vi "SUB-BLE SCAN.vi"(5 "Port-set 1":refnum<visa-resource-name>="COM8" caption="COM port") -> (0 "Device Name":string, 1 "Connection Status":T1={"MAC Address"="D9:2F:10:92:34:F2", "cnx handle"=0, "cnx flags"=5, "Address Type"=1, "Connection Interval (ms)"=15, "Timeout(ms)"=1000, "Latency"=0, "bonding handle"=255} {"Address Type" items=["Public", "Random"]}, 2 "Connected":bool)   [LabVIEW 2015]
doc: "Use this template to create an application that executes repeatedly until you click the Stop button. This template polls the state of the Stop button and does not use events. Use the Top-Level Application template (not available in the Base package) to create a single-loop application with event handling."
uses:
  Lib_Bled112 toolkit/type_def/connection_status_bundle.ctl
  Lib_Bled112 toolkit/type_def/address_type.ctl
panel:
  out "Discovery":bool
  out "conn flag":bool
  out "Handle table":string[][](array[string])
  out "Address Type":enum16{"Public", "Random"}(ring)=enum."Random"
  out "MAC Address":string="D9:2F:10:92:34:F2"
  in  "Cancel":bool
  in  "Connection":bool
  in  "새로 검색":bool
  out "Start Search":bool caption="검색 시작"
  out "Complete":bool
  in  "Device List":i32(listbox)=2
  out "Scanning":bool
  # "Device Select"
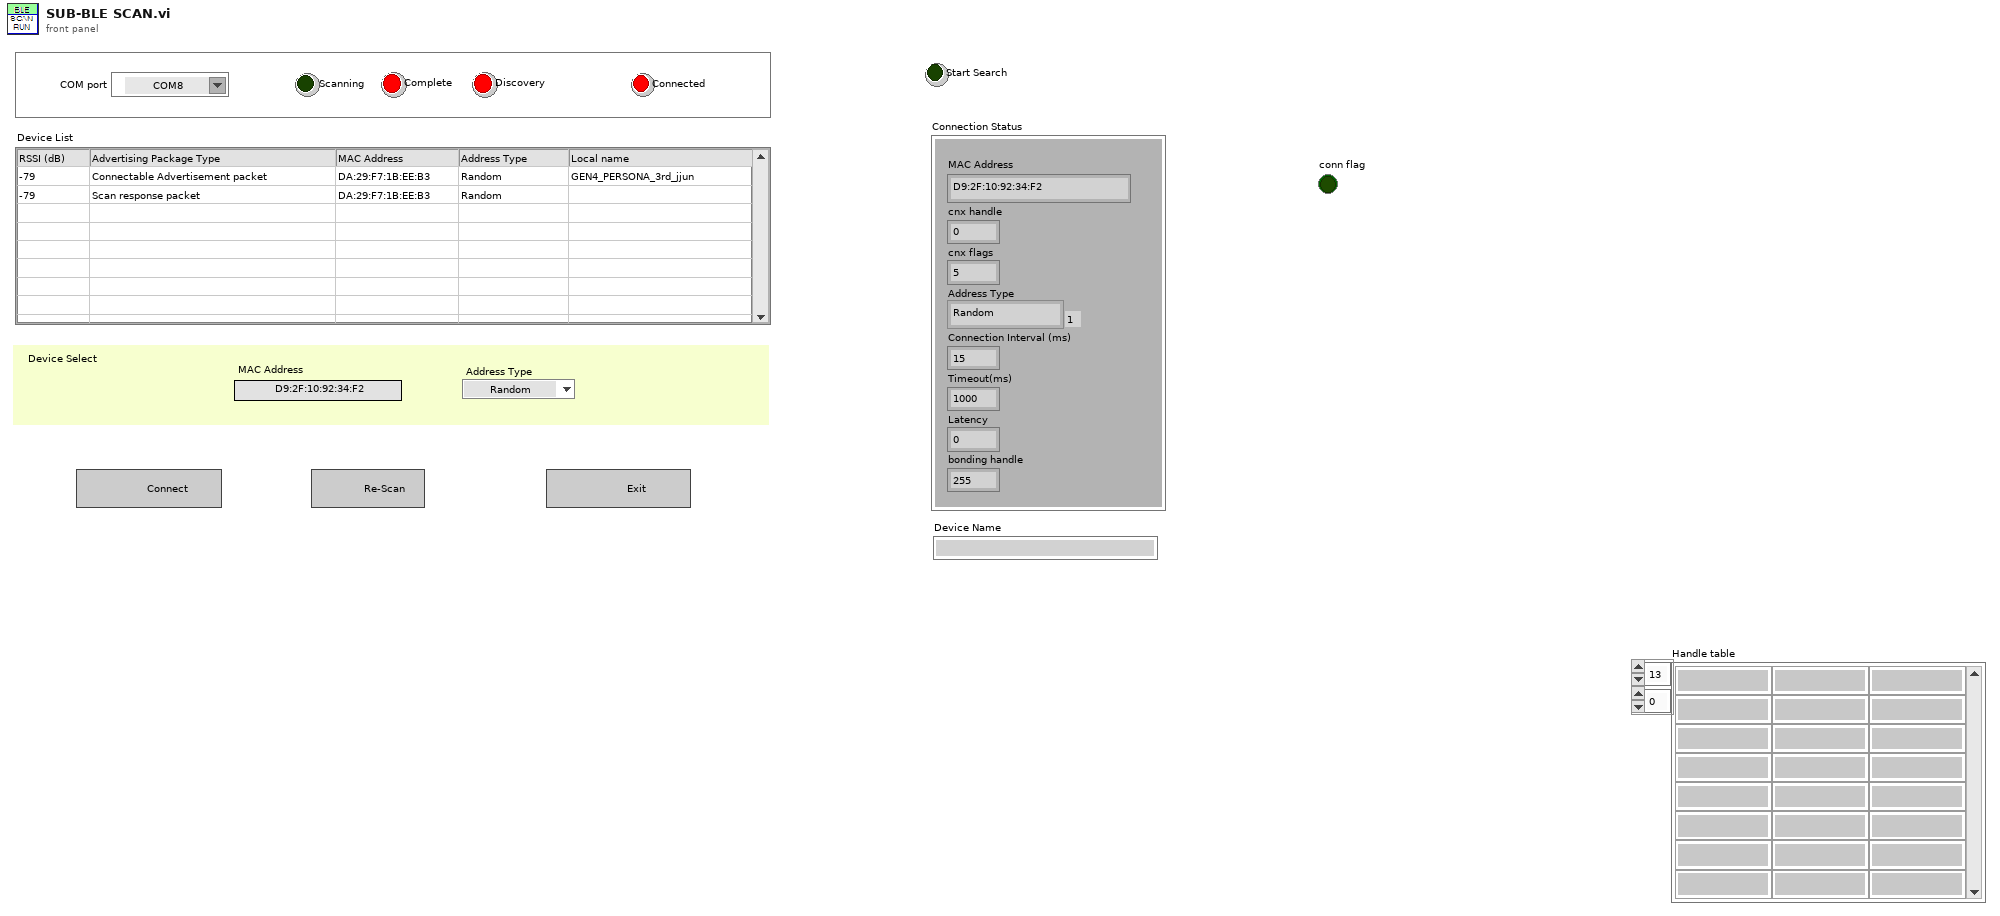
[diagram p1: front panel]
types:
  T1 = typedef "connection_status_bundle.ctl" = cluster{"MAC Address":string, "cnx handle":u8, "cnx flags":u8, "Address Type":T2, "Connection Interval (ms)":u16, "Timeout(ms)":u16, "Latency":u16, "bonding handle":u8}
  T2 = typedef "address_type.ctl" = u8
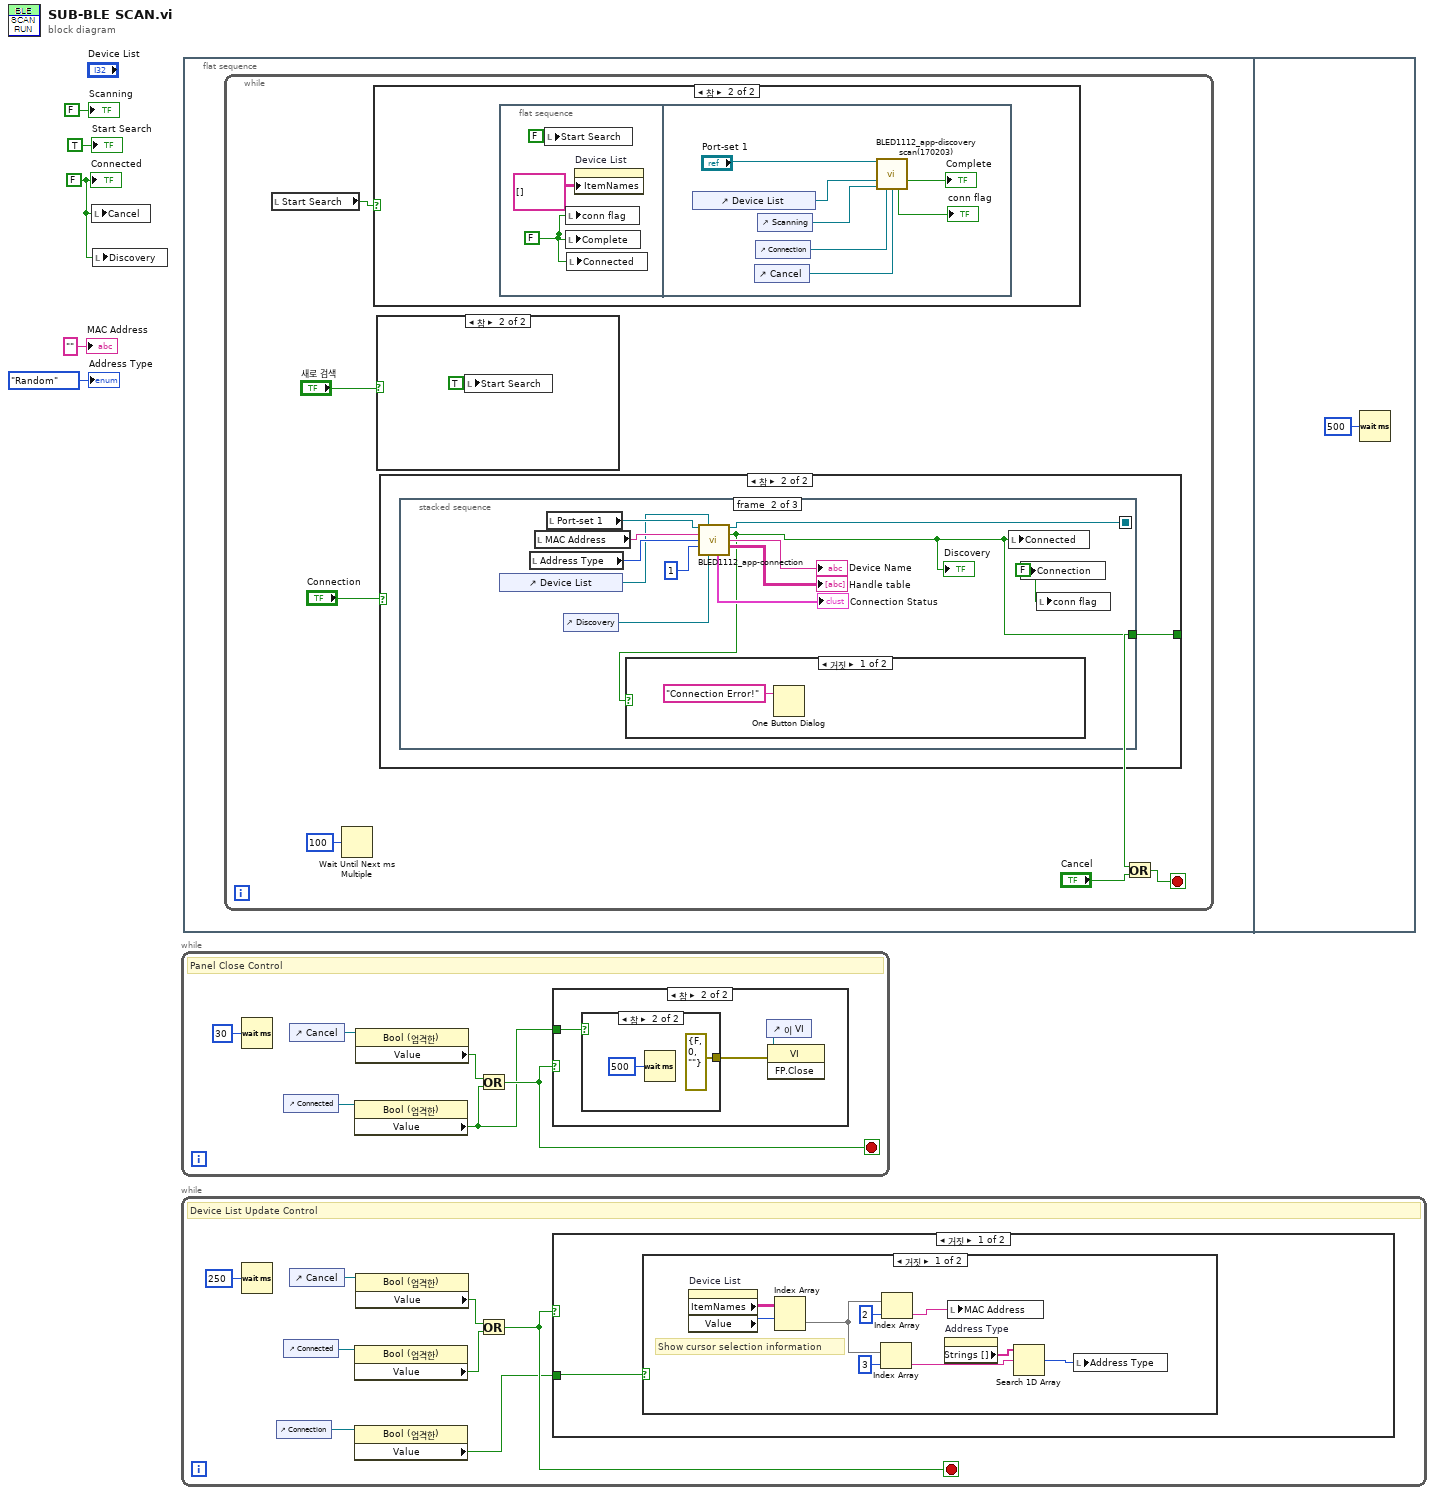
[diagram p0: block diagram]
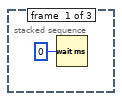
[diagram p7: hidden frame]
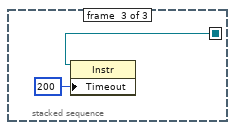
[diagram p9: hidden frame]
diagram:
  w1 = FALSE ("Connected")
  n1 = local write "Cancel"(w1) -> ()
  n2 = local write "Discovery"(w1) -> ()
  n3 = while {
    stop <- w7 stop-if-true
    # "Panel Close Control"
    n4 = Wait (ms)(milliseconds to wait=u32 30 ("대기 시간(ms)")) -> ()  [unwired: 1 out]
    n5 = control-ref of="Connected"() -> (w9:refnum<vi>)
    n6 = control-ref of="Cancel"() -> (w10:refnum<vi>)
    n7 = property class="Bool (엄격한)"(reference=w9) -> ("Value"=w6:bool)  [unwired: 1 in, 2 out]
    n8 = property class="Bool (엄격한)"(reference=w10) -> ("Value"=w8:bool)  [unwired: 1 in, 2 out]
    n9 = Or(x=w8, y=w6) -> (x .or. y?=w7:bool)
    n10 = case shown="참" w7 {
      tunnel: w6 -> [_ w13]
      frame False {
      }
      frame True {
        n11 = case shown="참" w13 {
          tunnel: [_ errorcluster {"status"=FALSE, "code"=0, "source"=""} ("에러 상수")] -> w12
          frame False {
          }
          frame True {
            n12 = Wait (ms)(milliseconds to wait=u32 500 ("대기 시간(ms)")) -> ()  [unwired: 1 out]
          }
        }
        n13 = control-ref of="이 VI"() -> (w14:refnum<vi>)
        n14 = invoke class="VI" method="FP.Close"(reference=w14, error in=w12) -> ()  [unwired: 1 in, 3 out]
      }
    }
  }
  n15 = while {
    stop <- w20 stop-if-true
    # "Device List Update Control"
    n16 = Wait (ms)(milliseconds to wait=u32 250 ("대기 시간(ms)")) -> ()  [unwired: 1 out]
    n17 = control-ref of="Connection"() -> (w18:refnum<vi>)
    n18 = control-ref of="Connected"() -> (w22:refnum<vi>)
    n19 = control-ref of="Cancel"() -> (w23:refnum<vi>)
    n20 = property class="Bool (엄격한)"(reference=w22) -> ("Value"=w19:bool)  [unwired: 1 in, 2 out]
    n21 = property class="Bool (엄격한)"(reference=w18) -> ("Value"=w17:bool)  [unwired: 1 in, 2 out]
    n22 = property class="Bool (엄격한)"(reference=w23) -> ("Value"=w21:bool)  [unwired: 1 in, 2 out]
    n23 = Or(x=w21, y=w19) -> (x .or. y?=w20:bool)
    n24 = case shown="거짓" w20 {
      tunnel: w17 -> [w25 _]
      frame False {
        n25 = case shown="거짓" w25 {
          frame False {
            # "Show cursor selection information"
            n26 = property on="Device List" class="MCListbox (엄격한)"() -> ("ItemNames"=w26:string[][], "Value"=w27:i32)  [unwired: 2 in, 2 out]
            n27 = Index Array(array=w26, index (row)=w27) -> (element=w31:string[])  [unwired: 1 in]
            n28 = Index Array(array=w31, index=3 ("인덱스")) -> (element=w32:string)
            n29 = Index Array(array=w31, index=2 ("인덱스")) -> (element=w29:string)
            n30 = property on="Address Type" class="Enum (엄격한)"() -> ("Strings []"=w34:string[])  [unwired: 2 in, 2 out]
            n31 = local write "MAC Address"(w29) -> ()
            n32 = Search 1D Array(1D array=w34, element=w32) -> (index of element=w33:i32)  [unwired: 1 in]
            n33 = local write "Address Type"(w33) -> ()
          }
          frame True {
          }
        }
      }
      frame True {
      }
    }
  }
  n34 = flat-sequence {
    frame #0 {
      n35 = while {
        stop <- w37 stop-if-true
        n36 = local read "Start Search"() -> (w41:bool)
        n37 = Wait Until Next ms Multiple(millisecond multiple=u32 100 ("ms 배수")) -> ()  [unwired: 1 out]
        n38 = case shown="참" w41 {
          frame False {
          }
          frame True {
            n39 = flat-sequence {
              frame #0 {
                w60 = FALSE ("검색 완료")
                n40 = local write "Start Search"(FALSE ("검색시작")) -> ()
                n41 = local write "conn flag"(w60) -> ()
                n42 = local write "Complete"(w60) -> ()
                n43 = local write "Connected"(w60) -> ()
                n44 = property on="Device List" class="MCListbox (엄격한)"("ItemNames"=string[][] [] ("아이템 이름")) -> ()  [unwired: 2 in, 2 out]
              }
              frame #1 {
                n45 = control-ref of="Device List"() -> (w66:refnum<vi>)
                n46 = control-ref of="Cancel"() -> (w64:refnum<vi>)
                n47 = control-ref of="Connection"() -> (w65:refnum<vi>)
                n48 = control-ref of="Scanning"() -> (w67:refnum<vi>)
                n49 = call "BLED1112_app-discovery scan(170203).vi"("COM in"="Port-set 1", "Device List"=w66, "LED ref"=w67, "Stop triger ref 1"=w65, "Stop triger ref 2"=w64) -> ("Scan success?"=→"Complete":bool, "Stop triger ref 1 out"=→"conn flag":bool)  [unwired: 6 in, 3 out]
              }
            }
          }
        }
        n50 = case shown="참" "새로 검색" {
          frame False {
          }
          frame True {
            n51 = local write "Start Search"(TRUE ("검색시작")) -> ()
          }
        }
        n52 = case shown="참" "Connection" {
          tunnel: [_ w42] -> w38
          frame False {
          }
          frame True {
            n53 = stacked-sequence {
              seq-local: [_ w44 _] -> [_ _ w58]
              tunnel: [_ w45 _] -> w42
              frame #0 {
                n54 = Wait (ms)(milliseconds to wait=u32 0 ("대기 시간(ms)")) -> ()  [unwired: 1 out]
              }
              frame #1 {
                w48 = FALSE ("연결")
                n55 = control-ref of="Device List"() -> (w47:refnum<vi>)
                n56 = local read "Address Type"() -> (w50:enum16{"Public", "Random"})
                n57 = local read "MAC Address"() -> (w51:string)
                n58 = local read "Port-set 1"() -> (w49:refnum<visa-resource-name>)
                n59 = control-ref of="Discovery"() -> (w46:refnum<vi>)
                n60 = call "BLED1112_app-connection.vi"("COM Bluegiga in"=w49, "Device List"=w47, "MAC Address"=w51, "Address Type"=w50, "Conn Try no"=1, "discovery"=w46) -> ("COM out"=w44:refnum<visa-resource-name>, "Connection Ok"=w45:bool, "Device Name"=→"Device Name":string, "Handle table"=→"Handle table":string[][], "Connection Status"=→"Connection Status":T1)  [unwired: 4 in, 1 out]
                "Discovery" <- w45
                n61 = case shown="거짓" w45 {
                  frame False {
                    n62 = One Button Dialog(message="Connection Error!" ("메시지")) -> ()  [unwired: 1 in, 1 out]
                  }
                  frame True {
                  }
                }
                n63 = local write "Connected"(w45) -> ()
                n64 = local write "Connection"(w48) -> ()
                n65 = local write "conn flag"(w48) -> ()
              }
              frame #2 {
                n66 = property class="Instr"(reference=w58, "Timeout"=u32 200 ("General Settings:Timeout Value")) -> ()  [unwired: 1 in, 2 out]
              }
            }
          }
        }
        n67 = Or(x=w38, y="Cancel") -> (x .or. y?=w37:bool)
      }
    }
    frame #1 {
      n68 = Wait (ms)(milliseconds to wait=u32 500 ("대기 시간(ms)")) -> ()  [unwired: 1 out]
    }
  }
  "Scanning" <- FALSE ("Scanning")
  "Start Search" <- TRUE ("검색시작")
  "Connected" <- w1
  "MAC Address" <- "" ("MAC Address")
  "Address Type" <- enum16{"Public", "Random"}."Random" ("Address Type")
